vi "PH_VacuumControl.write historical Data.vi"(0 "i ref in":refnum<vi>, 5 "error in":errorcluster) -> (14 "i ref out":refnum<vi>, 19 "error out":errorcluster)   [LabVIEW 2014, in "PH_VacuumControl.lvlib"]
uses:
  PH_VacuumControl.lvlib
  PH_Common/PH_Common.lvlib
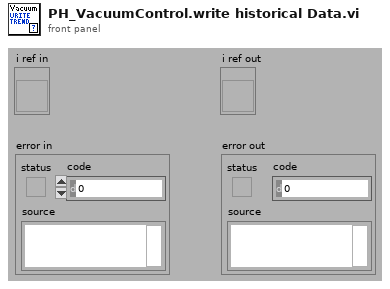
[diagram p1: front panel]
types:
  T1 = typedef "PH_VacuumControl.lvlib/PH_VacuumControl.i attribute.ctl" = cluster{"GUI Refs":cluster{"Exit":refnum<vi>, "Set Unit":refnum<vi>, "Device found":refnum<vi>, "Busy":refnum<vi>, "State":refnum<vi>, "Delete":refnum<vi>, "Channels":refnum<vi>, "Channel Name":refnum<vi>, "Trend":refnum<vi>, "Logarithmic":refnum<vi>, "Limit reached":refnum<vi>, "Channel Name 1 MT":refnum<vi>, "Channel Name 2 MT":refnum<vi>, "Trend MT":refnum<vi>, "Logarithmic MT":refnum<vi>, "Limit reached MT":refnum<vi>}, "Device found":bool, "Busy":bool, "Selected Unit":i32, "Channels [mbar]":T2, "Channel Names":cluster{"Channel 1":string, "Channel 2":string, "Channel 3":string, "Channel 4":string, "Channel 5":string, "Channel 6":string}, "Status":T3, "AGCxxx VISA Cluster":T4, "Instr Firmware Revision":string, "Service IDs Pressure":cluster{"Channel 1":i32, "Channel 2":i32, "Channel 3":i32, "Channel 4":i32, "Channel 5":i32, "Channel 6":i32}, "Service IDs Limits":cluster{"Channel 1":i32, "Channel 2":i32, "Channel 3":i32, "Channel 4":i32, "Channel 5":i32, "Channel 6":i32}, "Trend":cluster{"Start Point":timestamp, "Pressures [mbar] Channel 1":dbl[], "Pressures [mbar] Channel 2":dbl[], "Pressures [mbar] Channel 3":dbl[], "Pressures [mbar] Channel 4":dbl[], "Pressures [mbar] Channel 5":dbl[], "Pressures [mbar] Channel 6":dbl[], "Timebase [s]":i32[], "Trend Channel":u16, "Start Fit":dbl, "Trend Channel 1 MT":u16, "Trend Channel 2 MT":u16, "Start or continue Fit MT":dbl, "Continue or start Fit MT":dbl, "Datasets strored":i32, "Dataarray Size":i32}, "Running":bool}
  T2 = typedef "PH_VacuumControl.lvlib/PH_VacuumControl.Channels.ctl" = cluster{"Channel 1":dbl, "Channel 2":dbl, "Channel 3":dbl, "Channel 4":dbl, "Channel 5":dbl, "Channel 6":dbl, "Name Channel 1":string, "Name Channel 2":string, "Name Channel 3":string, "Name Channel 4":string, "Name Channel 5":string, "Name Channel 6":string, "Upper Limit":dbl, "Upper Limit 2":dbl, "Upper Limit 3":dbl, "Upper Limit 4":dbl, "Upper Limit 5":dbl, "Upper Limit 6":dbl}
  T3 = typedef "PH_StatusHandler.lvlib/PH_StatusHandler.Status.ctl" = i16
  T4 = typedef "AGCxxx - Driver.lvlib/AGCxxx VISA Control.ctl" = cluster{"VISA resource name":refnum<visa-resource-name>, "VISA Timeout Value (1000 ms)":u32, "Lock Timeout (1000 ms)":u32, "MAX Channel (6)":i32}
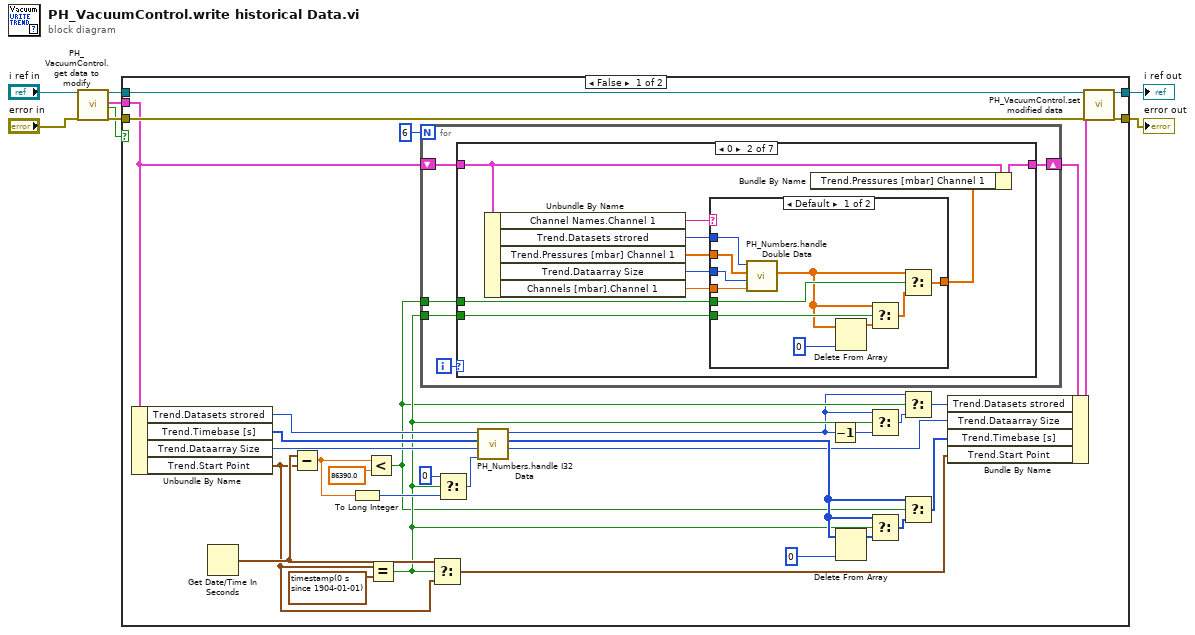
[diagram p0: block diagram]
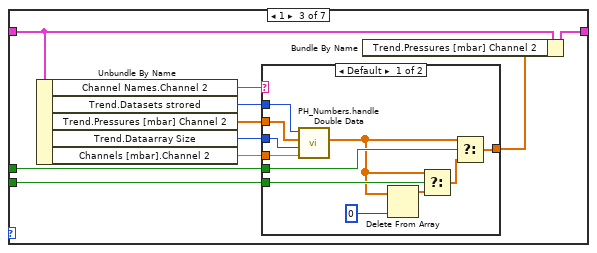
[diagram p4: hidden frame]
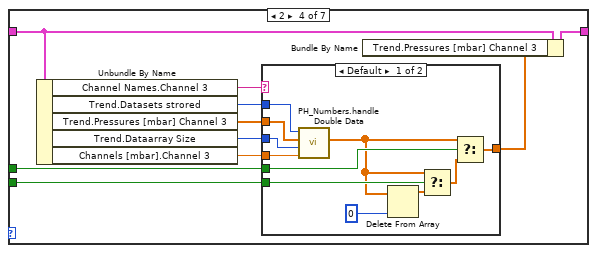
[diagram p6: hidden frame]
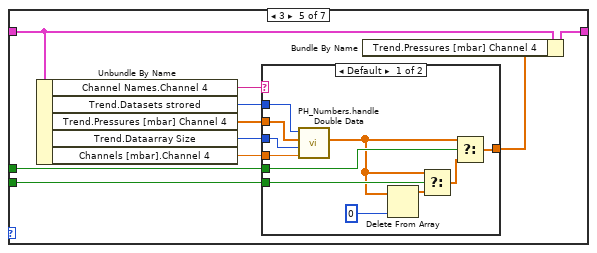
[diagram p8: hidden frame]
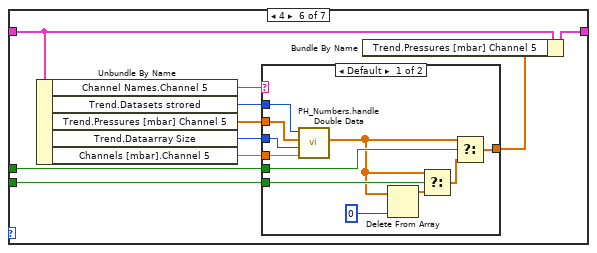
[diagram p10: hidden frame]
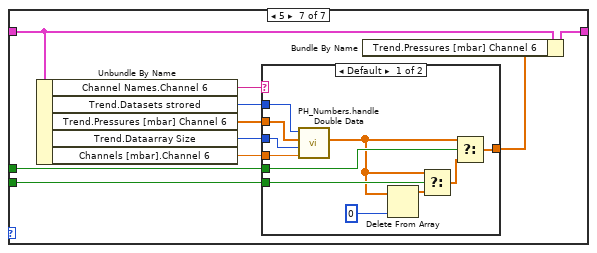
[diagram p12: hidden frame]
diagram:
  n1 = call "PH_VacuumControl.get data to modify.vi"("i ref in"="i ref in", "error in (no error)"="error in") -> ("i ref out"=w4:refnum<vi>, "i attribute"=w1:T1, "timed out"=w2:bool, "error out"=w7:errorcluster)  [unwired: 14 in]
  n2 = case shown="False" w2 {
    tunnel: w7 -> [w40 w179]
    tunnel: [w39 w179] -> w5
    tunnel: w4 -> [w38 w180]
    tunnel: [w37 w180] -> w3
    tunnel: w1 -> [w27 _]
    frame False {
      n3 = Unbundle By Name(w27) -> ("Trend.Datasets strored"=w17:i32, "Trend.Timebase [s]"=w20:i32[], "Trend.Dataarray Size"=w16:i32, "Trend.Start Point"=w22:timestamp)
      n4 = Get Date/Time In Seconds() -> (seconds since 1Jan1904=w34:timestamp)
      n5 = Subtract(x=w34, y=w22) -> (x-y=w32:dbl)
      n6 = To Long Integer(number=w32) -> (32bit integer=w30:i32)
      n7 = Less?(x=w32, y=86390.0) -> (x < y?=w12:bool)
      n8 = Equal?(x=w22, y=timestamp(0 s since 1904-01-01) ("Trend.Start Point")) -> (x = y?=w13:bool)
      n9 = for {
        N: 6 -> [_]
        tunnel: w12 -> [w42]
        tunnel: w13 -> [w41]
        shift-right: [w45] -> w26
        shift-left: w27 -> [w44]
        i -> [w43]
        n10 = case shown="0" w43 {
          tunnel: [w46 w56 w78 w100 w122 w144 w166] -> w45
          tunnel: w44 -> [w46 w55 w77 w99 w121 w143 w165]
          tunnel: w42 -> [_ w54 w76 w98 w120 w142 w164]
          tunnel: w41 -> [_ w53 w75 w97 w119 w141 w163]
          frame Default {
          }
          frame 0 {
            n11 = Unbundle By Name(w55) -> ("Channel Names.Channel 1"=w52:string, "Trend.Datasets strored"=w48:i32, "Trend.Pressures [mbar] Channel 1"=w50:dbl[], "Trend.Dataarray Size"=w47:i32, "Channels [mbar].Channel 1"=w49:dbl)
            n12 = case shown="Default" w52 {
              tunnel: w49 -> [w58 _]
              tunnel: w50 -> [w67 w68]
              tunnel: w54 -> [w64 _]
              tunnel: [w66 w68] -> w51
              tunnel: w53 -> [w63 _]
              tunnel: w48 -> [w59 _]
              tunnel: w47 -> [w57 _]
              frame Default {
                n13 = call "PH_Numbers.handle Double Data.vi"("New Datum"=w58, "Dataarray Size in"=w57, "Data in"=w67, "Datasets strored in"=w59) -> ("Data out"=w60:dbl[])  [unwired: 3 in, 2 out]
                n14 = Delete From Array(array=w60, index=0) -> (array with subset deleted=w62:dbl[])  [unwired: 1 in, 1 out]
                n15 = Select(t=w60, s=w63, f=w62) -> (s? t:f=w61:dbl[])
                n16 = Select(t=w60, s=w64, f=w61) -> (s? t:f=w66:dbl[])
              }
              frame "", "N/A" {
              }
            }
            n17 = Bundle By Name(cluster=w55, "Trend.Pressures [mbar] Channel 1"=w51) -> (w56:T1)
          }
          frame 1 {
            n18 = Unbundle By Name(w77) -> ("Channel Names.Channel 2"=w74:string, "Trend.Datasets strored"=w70:i32, "Trend.Pressures [mbar] Channel 2"=w72:dbl[], "Trend.Dataarray Size"=w69:i32, "Channels [mbar].Channel 2"=w71:dbl)
            n19 = case shown="Default" w74 {
              tunnel: w71 -> [w80 _]
              tunnel: w72 -> [w89 w90]
              tunnel: w76 -> [w86 _]
              tunnel: [w88 w90] -> w73
              tunnel: w75 -> [w85 _]
              tunnel: w70 -> [w81 _]
              tunnel: w69 -> [w79 _]
              frame Default {
                n20 = call "PH_Numbers.handle Double Data.vi"("New Datum"=w80, "Dataarray Size in"=w79, "Data in"=w89, "Datasets strored in"=w81) -> ("Data out"=w82:dbl[])  [unwired: 3 in, 2 out]
                n21 = Delete From Array(array=w82, index=0) -> (array with subset deleted=w84:dbl[])  [unwired: 1 in, 1 out]
                n22 = Select(t=w82, s=w85, f=w84) -> (s? t:f=w83:dbl[])
                n23 = Select(t=w82, s=w86, f=w83) -> (s? t:f=w88:dbl[])
              }
              frame "", "N/A" {
              }
            }
            n24 = Bundle By Name(cluster=w77, "Trend.Pressures [mbar] Channel 2"=w73) -> (w78:T1)
          }
          frame 2 {
            n25 = Unbundle By Name(w99) -> ("Channel Names.Channel 3"=w96:string, "Trend.Datasets strored"=w92:i32, "Trend.Pressures [mbar] Channel 3"=w94:dbl[], "Trend.Dataarray Size"=w91:i32, "Channels [mbar].Channel 3"=w93:dbl)
            n26 = case shown="Default" w96 {
              tunnel: w93 -> [w102 _]
              tunnel: w94 -> [w111 w112]
              tunnel: w98 -> [w108 _]
              tunnel: [w110 w112] -> w95
              tunnel: w97 -> [w107 _]
              tunnel: w92 -> [w103 _]
              tunnel: w91 -> [w101 _]
              frame Default {
                n27 = call "PH_Numbers.handle Double Data.vi"("New Datum"=w102, "Dataarray Size in"=w101, "Data in"=w111, "Datasets strored in"=w103) -> ("Data out"=w104:dbl[])  [unwired: 3 in, 2 out]
                n28 = Delete From Array(array=w104, index=0) -> (array with subset deleted=w106:dbl[])  [unwired: 1 in, 1 out]
                n29 = Select(t=w104, s=w107, f=w106) -> (s? t:f=w105:dbl[])
                n30 = Select(t=w104, s=w108, f=w105) -> (s? t:f=w110:dbl[])
              }
              frame "", "N/A" {
              }
            }
            n31 = Bundle By Name(cluster=w99, "Trend.Pressures [mbar] Channel 3"=w95) -> (w100:T1)
          }
          frame 3 {
            n32 = Unbundle By Name(w121) -> ("Channel Names.Channel 4"=w118:string, "Trend.Datasets strored"=w114:i32, "Trend.Pressures [mbar] Channel 4"=w116:dbl[], "Trend.Dataarray Size"=w113:i32, "Channels [mbar].Channel 4"=w115:dbl)
            n33 = case shown="Default" w118 {
              tunnel: w115 -> [w124 _]
              tunnel: w116 -> [w133 w134]
              tunnel: w120 -> [w130 _]
              tunnel: [w132 w134] -> w117
              tunnel: w119 -> [w129 _]
              tunnel: w114 -> [w125 _]
              tunnel: w113 -> [w123 _]
              frame Default {
                n34 = call "PH_Numbers.handle Double Data.vi"("New Datum"=w124, "Dataarray Size in"=w123, "Data in"=w133, "Datasets strored in"=w125) -> ("Data out"=w126:dbl[])  [unwired: 3 in, 2 out]
                n35 = Delete From Array(array=w126, index=0) -> (array with subset deleted=w128:dbl[])  [unwired: 1 in, 1 out]
                n36 = Select(t=w126, s=w129, f=w128) -> (s? t:f=w127:dbl[])
                n37 = Select(t=w126, s=w130, f=w127) -> (s? t:f=w132:dbl[])
              }
              frame "", "N/A" {
              }
            }
            n38 = Bundle By Name(cluster=w121, "Trend.Pressures [mbar] Channel 4"=w117) -> (w122:T1)
          }
          frame 4 {
            n39 = Unbundle By Name(w143) -> ("Channel Names.Channel 5"=w140:string, "Trend.Datasets strored"=w136:i32, "Trend.Pressures [mbar] Channel 5"=w138:dbl[], "Trend.Dataarray Size"=w135:i32, "Channels [mbar].Channel 5"=w137:dbl)
            n40 = case shown="Default" w140 {
              tunnel: w137 -> [w146 _]
              tunnel: w138 -> [w155 w156]
              tunnel: w142 -> [w152 _]
              tunnel: [w154 w156] -> w139
              tunnel: w141 -> [w151 _]
              tunnel: w136 -> [w147 _]
              tunnel: w135 -> [w145 _]
              frame Default {
                n41 = call "PH_Numbers.handle Double Data.vi"("New Datum"=w146, "Dataarray Size in"=w145, "Data in"=w155, "Datasets strored in"=w147) -> ("Data out"=w148:dbl[])  [unwired: 3 in, 2 out]
                n42 = Delete From Array(array=w148, index=0) -> (array with subset deleted=w150:dbl[])  [unwired: 1 in, 1 out]
                n43 = Select(t=w148, s=w151, f=w150) -> (s? t:f=w149:dbl[])
                n44 = Select(t=w148, s=w152, f=w149) -> (s? t:f=w154:dbl[])
              }
              frame "", "N/A" {
              }
            }
            n45 = Bundle By Name(cluster=w143, "Trend.Pressures [mbar] Channel 5"=w139) -> (w144:T1)
          }
          frame 5 {
            n46 = Unbundle By Name(w165) -> ("Channel Names.Channel 6"=w162:string, "Trend.Datasets strored"=w158:i32, "Trend.Pressures [mbar] Channel 6"=w160:dbl[], "Trend.Dataarray Size"=w157:i32, "Channels [mbar].Channel 6"=w159:dbl)
            n47 = case shown="Default" w162 {
              tunnel: w159 -> [w168 _]
              tunnel: w160 -> [w177 w178]
              tunnel: w164 -> [w174 _]
              tunnel: [w176 w178] -> w161
              tunnel: w163 -> [w173 _]
              tunnel: w158 -> [w169 _]
              tunnel: w157 -> [w167 _]
              frame Default {
                n48 = call "PH_Numbers.handle Double Data.vi"("New Datum"=w168, "Dataarray Size in"=w167, "Data in"=w177, "Datasets strored in"=w169) -> ("Data out"=w170:dbl[])  [unwired: 3 in, 2 out]
                n49 = Delete From Array(array=w170, index=0) -> (array with subset deleted=w172:dbl[])  [unwired: 1 in, 1 out]
                n50 = Select(t=w170, s=w173, f=w172) -> (s? t:f=w171:dbl[])
                n51 = Select(t=w170, s=w174, f=w171) -> (s? t:f=w176:dbl[])
              }
              frame "", "N/A" {
              }
            }
            n52 = Bundle By Name(cluster=w165, "Trend.Pressures [mbar] Channel 6"=w161) -> (w166:T1)
          }
        }
      }
      n53 = Select(t=w34, s=w13, f=w22) -> (s? t:f=w23:timestamp)
      n54 = Select(t=0, s=w13, f=w30) -> (s? t:f=w18:i32)
      n55 = call "PH_Numbers.handle I32 Data.vi"("New Datum"=w18, "Dataarray Size in"=w16, "Data in"=w20, "Datasets strored in"=w17) -> ("Dataarray Size out"=w15:i32, "Data out"=w19:i32[], "Datasets strored out"=w10:i32)  [unwired: 3 in]
      n56 = Decrement(x=w10) -> (x-1=w9:i32)
      n57 = Delete From Array(array=w19, index=0) -> (array with subset deleted=w29:i32[])  [unwired: 1 in, 1 out]
      n58 = Select(t=w10, s=w13, f=w9) -> (s? t:f=w14:i32)
      n59 = Select(t=w19, s=w13, f=w29) -> (s? t:f=w28:i32[])
      n60 = Select(t=w10, s=w12, f=w14) -> (s? t:f=w11:i32)
      n61 = Select(t=w19, s=w12, f=w28) -> (s? t:f=w24:i32[])
      n62 = Bundle By Name(cluster=w26, "Trend.Datasets strored"=w11, "Trend.Dataarray Size"=w15, "Trend.Timebase [s]"=w24, "Trend.Start Point"=w23) -> (w25:T1)
      n63 = call "PH_VacuumControl.set modified data.vi"("i ref in"=w38, "i attribute"=w25, "error in (no error)"=w40) -> ("i ref out"=w37:refnum<vi>, "error out"=w39:errorcluster)  [unwired: 15 in]
    }
    frame True {
    }
  }
  "i ref out" <- w3
  "error out" <- w5
